vi "Flow.vi"() -> ()   [LabVIEW 2018]
uses:
  <vilib>/Utility/config.llb/Config Data RefNum.ctl
  <vilib>/Utility/sysdir.llb/System Directory Type.ctl
  modules/Serial - XON-XOFF Characters.ctl
  modules/Serial - ASCII Characters.ctl
  modules/Serial - Settings.ctl
  <vilib>/Utility/config.llb/Read Key (String).vi
  <vilib>/Utility/config.llb/Write Key (String).vi
  <vilib>/Utility/config.llb/NI_LVConfig.lvlib
panel:
  out "error out":errorcluster
  out "queue":refnum<queue>
  out "Driver Status":errorcluster
  in  "Marker":string="start_marker"
  out "State":enum16{"Connect", "Acquire", "Standby"}(ring)=enum."Standby"
  in  "S4":dbl[](array[numeric])=[0.0, 0.0, 0.0, 0.0]
  in  "S3":dbl[](array[numeric])=[0.0, 0.0, 0.0, 0.0]
  in  "S2":dbl[](array[numeric])=[0.0, 0.0, 0.0, 0.0]
  in  "S1":dbl[](array[numeric])=[0.0, 0.0, 0.0, 0.0]
  out "System Path":path
  out "dStruct":string[](array[string])
  out "TDMS":refnum<k34>
  in  "?":enum32{"Overview", "Flow vs. Pressure Char"}(tab)
  out "Waveform Chart":dbl(graph)
  out "Flow vs Pressure":cluster{"X":dbl[], "Y":dbl[]}[](graph)
  in  "Enable":bool=TRUE
  in  "Tab Control":enum32{"Connection", "Diagnostic"}(tab)
  in  "add marker":bool
  in  "Record":bool
  in  "New File":bool
  in  "markerString":string
  in  "Folder":path
  in  "File Name":string="database"
  in  "VISA":refnum<visa-resource-name>="COM4"
  in  "EXIT":bool
  in  "Connect":bool
  out "Latency:":dbl
  out "Terminal":string
  in  "Command Terminal":string
  out "Serial Settings:Number of Bytes at Serial Port":u32
  out "Device:":string
  out "Battery Voltage":dbl(slide) scale=3.2..4.2 scale format="%#_2g"
  out "Error Out":errorcluster
  out "Config File":T1
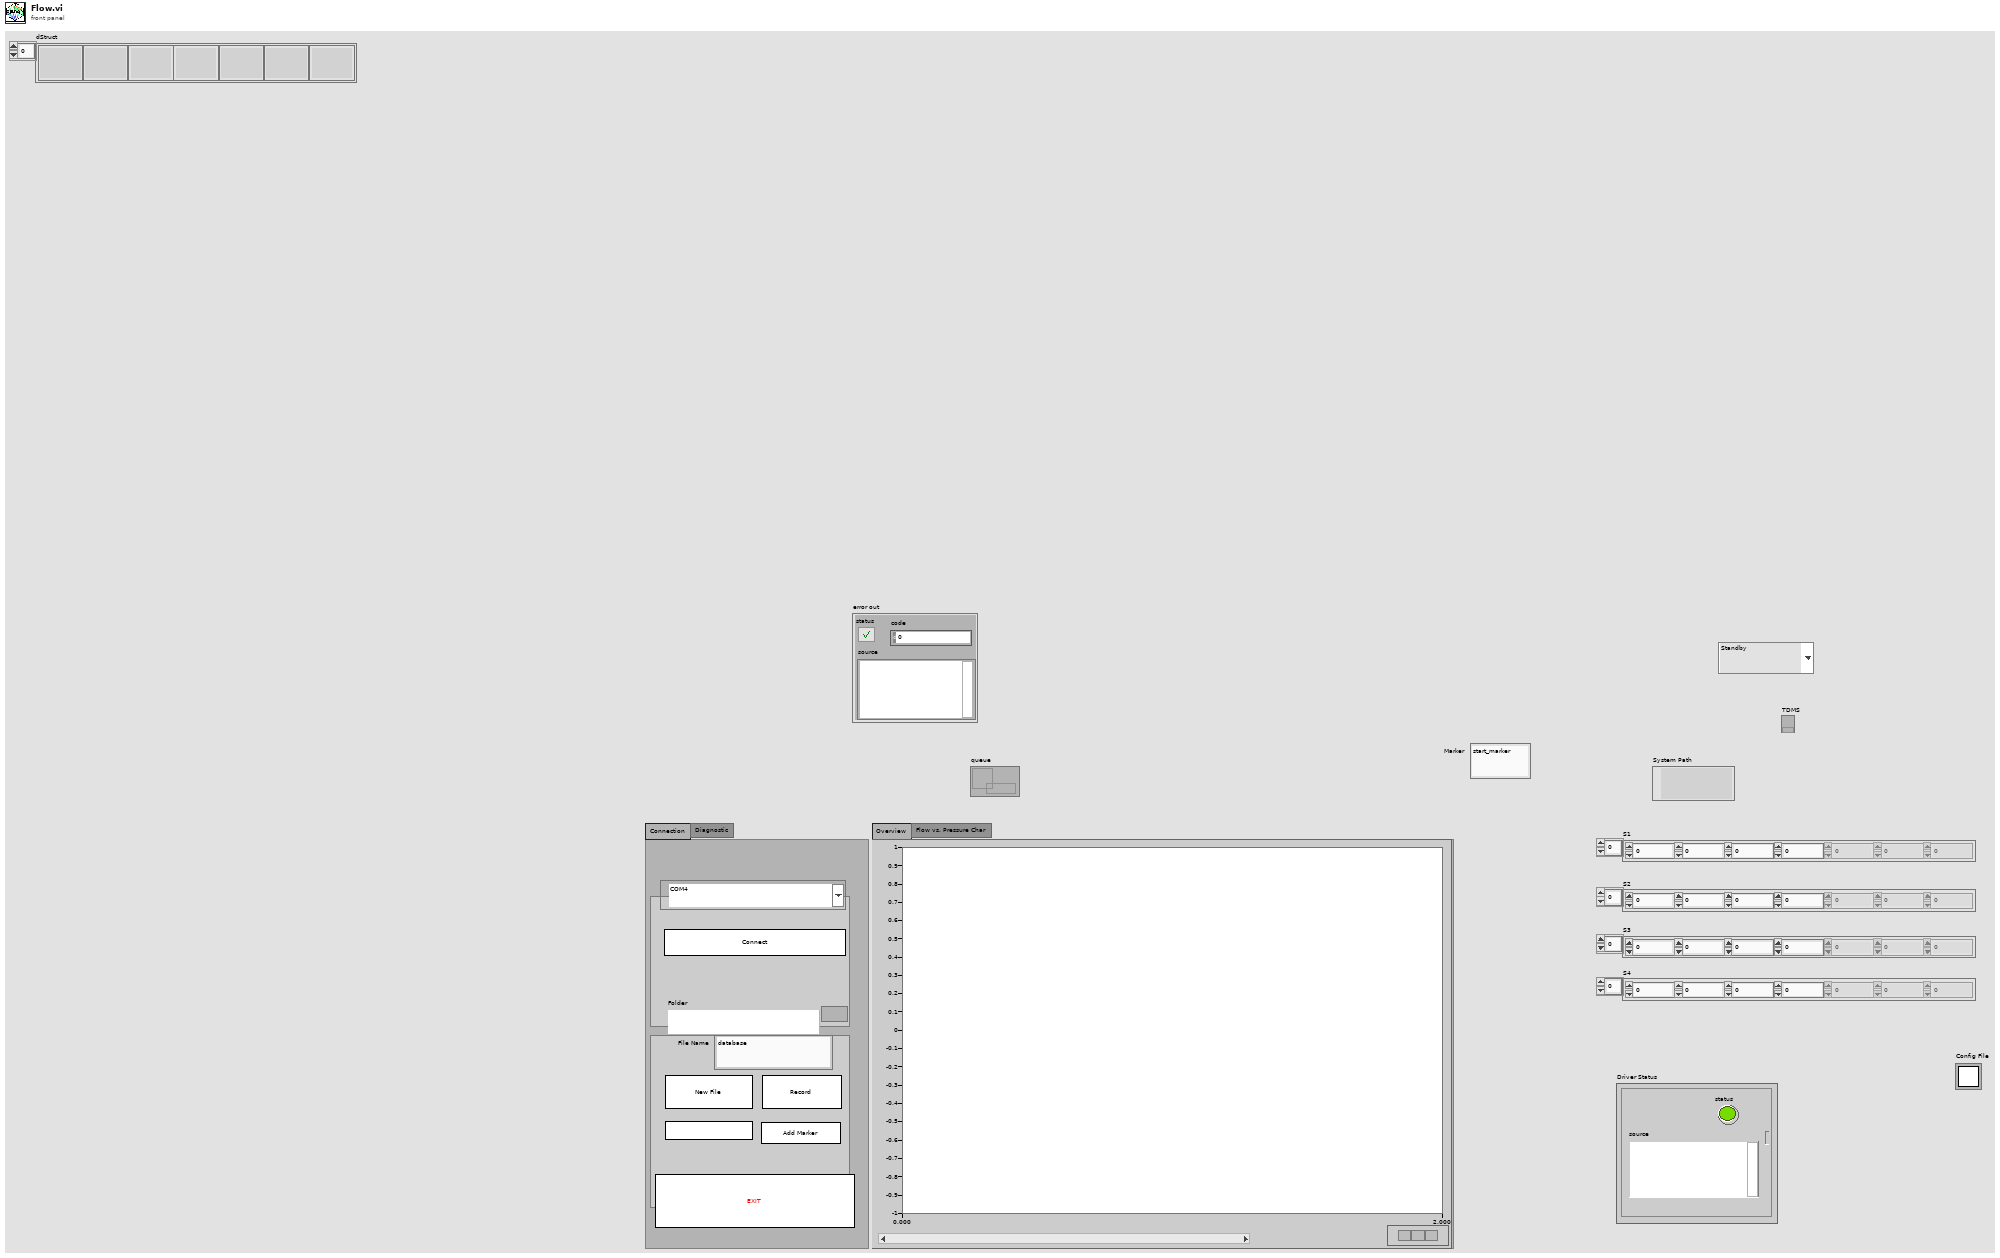
[diagram p1: front panel]
types:
  T1 = typedef "NI_LVConfig.lvlib/Config Data RefNum.ctl" = refnum<k1>
  T2 = cluster{"Dynamic Data Type":dynamicdata, string[]}
  T3 = typedef "System Directory Type.ctl" = i32
  T4 = typedef "Serial - Settings.ctl" = cluster{"baud rate":u32, "data bits":u16, "parity":enum16{"None", "Odd", "Even", "Mark", "Space"}, "stop bits":u16, "flow control":u16}
  T5 = typedef "Serial - XON-XOFF Characters.ctl" = cluster{"XON":T6, "XOFF":T6}
  T6 = typedef "Serial - ASCII Characters.ctl" = enum16{"NUL", "SOH", "STX", "ETX", "EOT", "ENQ", "ACK", "BEL", "BS", "HT", "LF", "VT", "FF", "CR", "SO", "SI", "DLE", "DC1", "DC2", "DC3", "DC4", "NAK", "SYN", "ETB", "CAN", "EM", "SUB", "ESC", "FS", "GS", "RS", "US", "SP", "!", "\"", "#", "$", "%", "&", "'", "(", ")", "*", "+", ",", "- (-)", ".", "/", "0", "1", "2", "3", "4", "5", "6", "7", "8", "9", ":", ";", "<", "=", ">", "?", "@", "A", "B", "C", "D", "E", "F", "G", "H", "I", "J", "K", "L", "M", "N", "O", "P", "Q", "R", "S", "T", "U", "V", "W", "X", "Y", "Z", "[", "\\", "]", "^", "_", "`", "a", "b", "c", "d", "e", "f", "g", "h", "i", "j", "k", "l", "m", "n", "o", "p", "q", "r", "s", "t", "u", "v", "w", "x", "y", "z", "{", "|", "}", "~"}
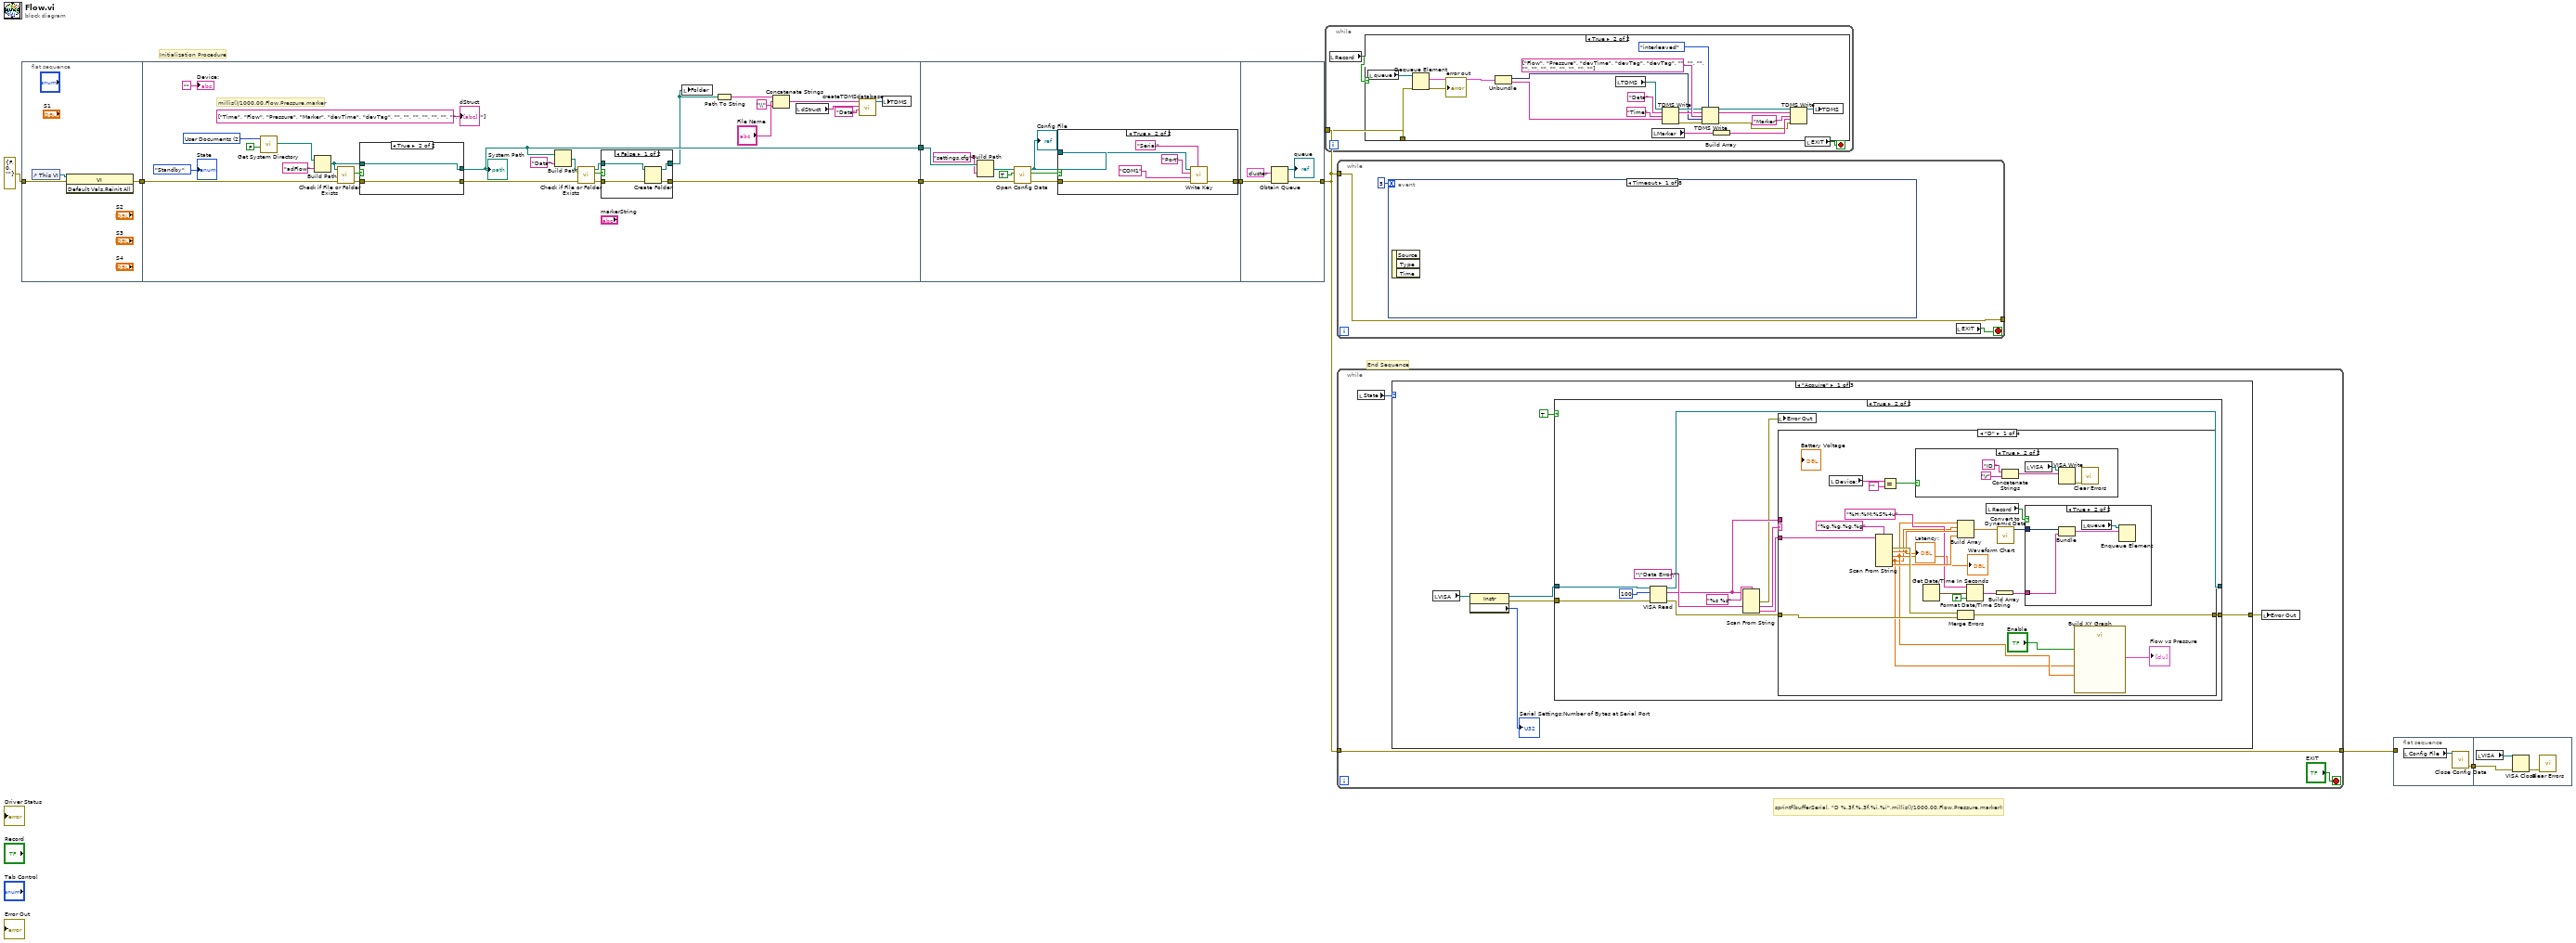
[diagram p0: block diagram]
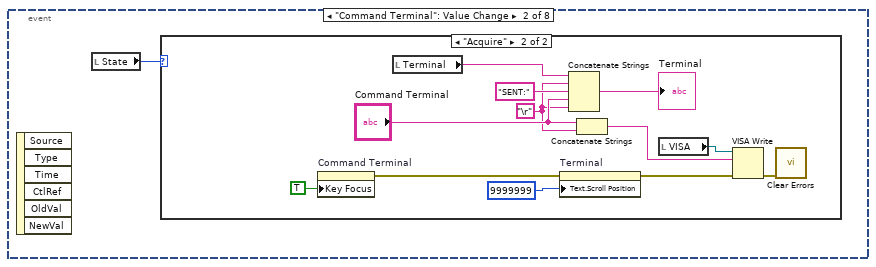
[diagram p3: hidden frame]
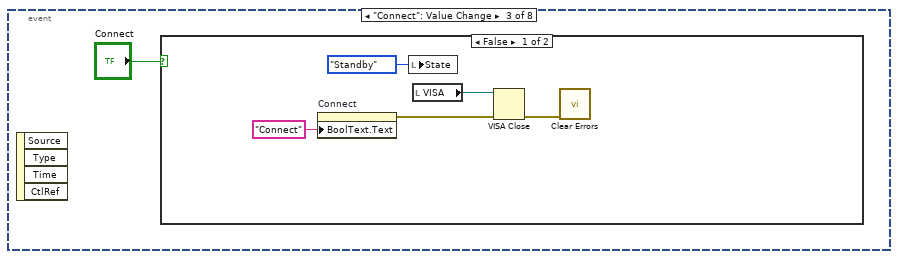
[diagram p5: hidden frame]
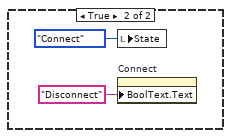
[diagram p6: hidden frame]
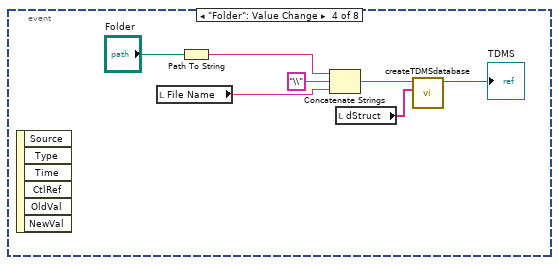
[diagram p7: hidden frame]
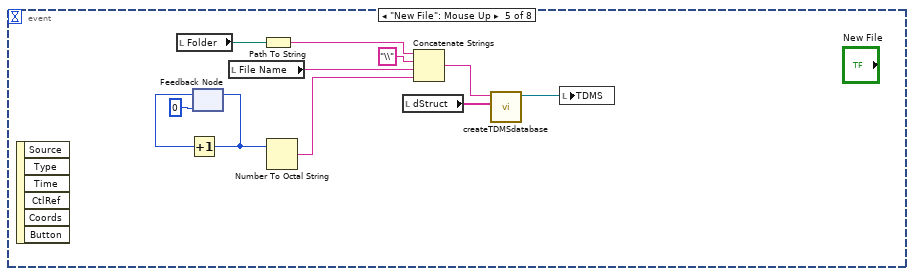
[diagram p8: hidden frame]
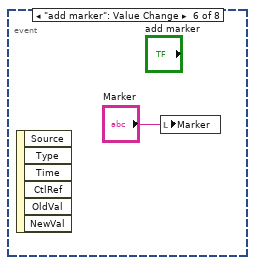
[diagram p9: hidden frame]
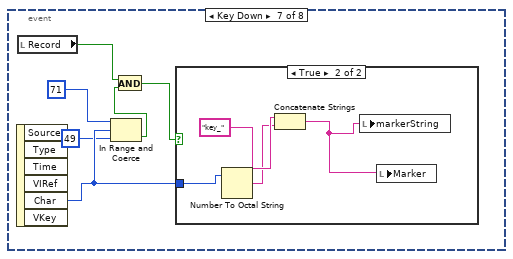
[diagram p10: hidden frame]
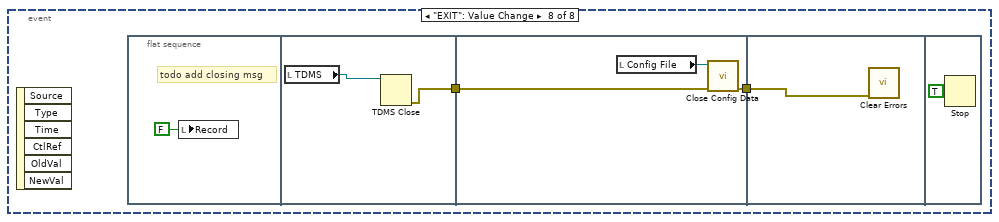
[diagram p12: hidden frame]
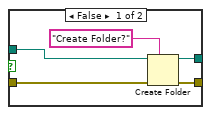
[diagram p14: hidden frame]
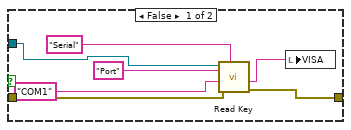
[diagram p15: hidden frame]
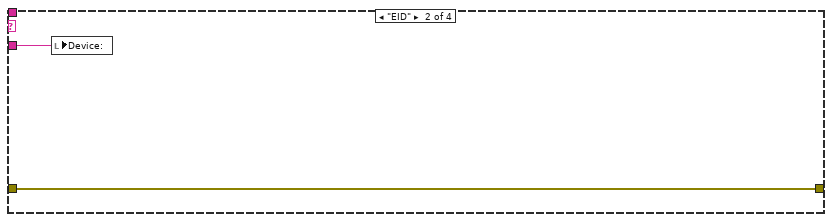
[diagram p19: hidden frame]
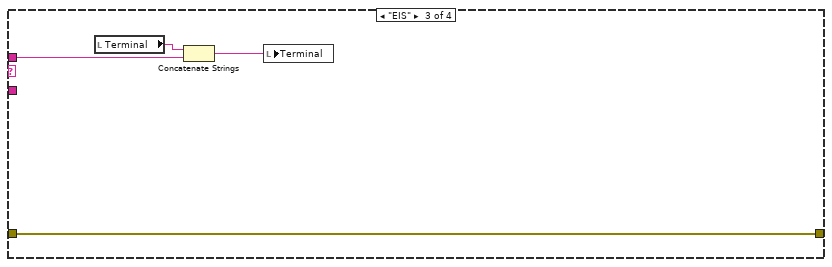
[diagram p20: hidden frame]
diagram:
  # "sprintf(bufferSerial, \"D %.3f,%.3f,%i,%i\",millis()/1000.00,Flow,Pressure,marker);"
  # "End Sequence"
  # "Initialization Procedure"
  n1 = flat-sequence {
    tunnel: errorcluster {"status"=FALSE, "code"=0, "source"=""} ("error in (no error)") -> [w10]
    tunnel: [w9] -> w5
    tunnel: [w28] -> w7
    tunnel: [w25] -> w6
    tunnel: w5 -> [w34]
    tunnel: w7 -> [w58]
    tunnel: w6 -> [w60]
    tunnel: [w52] -> w3
    tunnel: [w75] -> w2
    tunnel: w3 -> [w77]
    frame #0 {
      n2 = control-ref of="This VI"() -> (w11:refnum<vi>)
      n3 = invoke class="VI" method="Default Vals.Reinit All"(reference=w11, error in=w10) -> (error out=w9:errorcluster)  [unwired: 1 in, 2 out]
    }
    frame #1 {
      w37 = T3 2 items=["User Home"=0, "User Desktop"=1, "User Documents"=2, "User Application Data"=3, "User Preferences"=4, "User Temporary"=5, "Public Documents"=6, "Public Application Data"=7, "Public Preferences"=8, "Public Cache"=13, "System Core Libraries"=9, "System Installed Libraries"=10, "Application Files"=11, "Boot Volume Root"=12] ("system directory type")
      # "millis()/1000.00,Flow,Pressure,marker"
      n4 = call <vilib>:"Get System Directory.vi"("create directory if not found? (F)"=FALSE, "system directory type"=w37) -> ("system directory"=w36:path)  [unwired: 9 in]
      n5 = Build Path(base path=w36, name or relative path="adFlow") -> (appended path=w32:path)
      n6 = call <vilib>:"Check if File or Folder Exists.vi"("error in (no error)"=w34, "path"=w32) -> ("error out"=w31:errorcluster, "file or folder exists?"=w33:bool)  [unwired: 7 in, 1 out]
      n7 = case shown="True" w33 {
        tunnel: w32 -> [w49 w51]
        tunnel: w31 -> [w48 w50]
        tunnel: [w46 w51] -> w28
        tunnel: [w45 w50] -> w27
        frame False {
          n8 = Create Folder(prompt (Create Folder)="Create Folder?", path (use dialog)=w49, error in=w48) -> (created path=w46:path, error out=w45:errorcluster)  [unwired: 1 out]
        }
        frame True {
        }
      }
      "System Path" <- w28
      n9 = Build Path(base path=w28, name or relative path="Data") -> (appended path=w29:path)
      n10 = call <vilib>:"Check if File or Folder Exists.vi"("error in (no error)"=w27, "path"=w29) -> ("error out"=w26:errorcluster, "file or folder exists?"=w24:bool, "dup path"=w23:path)  [unwired: 7 in]
      n11 = case shown="False" w24 {
        tunnel: [w41 w44] -> w25
        tunnel: w26 -> [w42 w44]
        tunnel: w23 -> [w40 w43]
        tunnel: [w39 w43] -> w21
        frame False {
          n12 = Create Folder(path (use dialog)=w40, error in=w42) -> (created path=w39:path, error out=w41:errorcluster)  [unwired: 1 in, 1 out]
        }
        frame True {
        }
      }
      n13 = local write "Folder"(w21) -> ()
      n14 = Path To String(path=w21) -> (string=w16:string)
      n15 = Concatenate Strings(w16, "\\" ("string"), "File Name") -> (w20:string)
      n16 = local read "dStruct"() -> (w19:string[])
      n17 = call "createTDMSdatabase.vi"("group name in (Untitled)"="Data", "channel name(s) in (Untitled)"=w19, "String"=w20) -> ("Refnum out"=w22:refnum<k34>)  [unwired: 8 in]
      n18 = local write "TDMS"(w22) -> ()
      "dStruct" <- string[] ["Time", "Flow", "Pressure", "Marker", "devTime", "devTag", "", "", "", "", "", "", "", "", "", ""] ("Channel Names")
      "Device:" <- ""
      "State" <- enum16{"Connect", "Acquire", "Standby"}."Standby" ("State")
    }
    frame #2 {
      n19 = Build Path(base path=w58, name or relative path="settings.cfg") -> (appended path=w56:path)
      n20 = call <vilib>:"Open Config Data.vi"("error in (no error)"=w60, "create file if necessary (T)"=TRUE, "configuration file path"=w56) -> ("error out"=w53:errorcluster, "file created?"=w55:bool, "refnum"=w54:T1)  [unwired: 6 in]
      "Config File" <- w54
      n21 = case shown="True" w55 {
        tunnel: w54 -> [w61 w73]
        tunnel: w53 -> [w63 w72]
        tunnel: [w62 w71] -> w52
        frame False {
          n22 = call-poly <vilib>:"Read Key.vi"("section"="Serial", "error in (no error)"=w63, "default value"="COM1" ("key"), "key"="Port", "refnum"=w61) -> ("error out"=w62:errorcluster, "value"=w67:string)  [unwired: 3 in, 2 out]
          n23 = local write "VISA"(w67) -> ()
        }
        frame True {
          n24 = call-poly <vilib>:"Write Key.vi"("section"="Serial", "error in (no error)"=w72, "value"="COM1" ("key"), "key"="Port", "refnum"=w73) -> ("error out"=w71:errorcluster)  [unwired: 4 in, 2 out]
        }
      }
    }
    frame #3 {
      n25 = Obtain Queue(element data type=T2 {"Dynamic Data Type"=[{"t0"=timestamp(0 s since 1904-01-01), "dt"=1.0, "Y"=[0.0, 0.0, 0.0, 0.0]}, {"t0"=timestamp(3629832558.8844056 s since 1904-01-01), "dt"=1.0, "Y"=[0.0]}, {"t0"=timestamp(3629832558.8844056 s since 1904-01-01), "dt"=1.0, "Y"=[1628.381]}, {"t0"=timestamp(3629832558.8844056 s since 1904-01-01), "dt"=1.0, "Y"=[0.0]}], ["0:00:00.0000"]} ("queue cluster"), error in (no error)=w77) -> (queue out=→"queue":refnum<queue>, error out=w75:errorcluster)  [unwired: 3 in, 1 out]
    }
  }
  n26 = while {
    tunnel: w2 -> [w80]
    stop <- w79 stop-if-true
    n27 = local read "Record"() -> (w78:bool)
    n28 = case shown="True" w78 {
      tunnel: w80 -> [_ w100]
      frame False {
      }
      frame True {
        n29 = local read "queue"() -> (w101:refnum<queue>)
        n30 = Dequeue Element(queue=w101, error in (no error)=w100) -> (element=w99:T2, error out=→"error out":errorcluster)  [unwired: 1 in, 2 out]
        n31 = Unbundle(w99) -> ("Dynamic Data Type"=w83:dynamicdata, w84:string[])
        n32 = local read "TDMS"() -> (w92:refnum<k34>)
        n33 = local read "Marker"() -> (w93:string)
        n34 = TDMS Write(0:w92, 5:"Data" ("group name in (Untitled)"), 7:"Time" ("group name in (Untitled)"), 9:w84) -> (4:w88:refnum<k34>, 6:w89:string, 15:w90:errorcluster)  [unwired: 2 in, 1 out]
        n35 = TDMS Write(0:w88, 1:enum16{"decimated", "interleaved"}."interleaved" ("data layout (0:decimated)"), 5:w89, 7:string[] ["Flow", "Pressure", "devTime", "devTag", "devTag", "", "", "", "", "", "", "", "", "", "", ""] ("Channel Names"), 9:w83, 11:w90) -> (4:w86:refnum<k34>, 6:w85:string, 15:w81:errorcluster)  [unwired: 1 out]
        n36 = Build Array(w93) -> (w94:string[])
        n37 = TDMS Write(0:w86, 5:w85, 7:"Marker" ("channel name(s) in (Untitled)"), 9:w94, 11:w81) -> (4:w97:refnum<k34>)  [unwired: 1 in, 3 out]
        n38 = local write "TDMS"(w97) -> ()
      }
    }
    n39 = local read "EXIT"() -> (w79:bool)
  }
  n40 = while {
    tunnel: w2 -> [w103]
    tunnel: [w103] -> _
    stop <- w104 stop-if-true
    n41 = event shown="[0] Timeout" {
      selector: _ -> [_ _ _ _ _ _ _ _]
      dyn-events: _ -> [_ _ _ _ _ _ _ _]
      timeout: 5 -> [_ _ _ _ _ _ _ _]
      event Timeout {
        n42 = event-data() -> ()  [unwired: 1 in, 3 out]
      }
      event "Command Terminal": Value Change {
        n43 = event-data() -> ()  [unwired: 1 in, 6 out]
        n44 = local read "State"() -> (w105:enum16{"Connect", "Acquire", "Standby"})
        n45 = case shown="\"Acquire\"" w105 {
          frame "Connect", Default {
          }
          frame "Acquire" {
            w108 = "\r"
            n46 = property on="Command Terminal" class="Str"("Key Focus"=TRUE) -> (error out=w113:errorcluster)  [unwired: 2 in, 1 out]
            n47 = local read "Terminal"() -> (w117:string)
            n48 = property on="Terminal" class="Str"(error in=w113, "Text.Scroll Position"=u32 9999999) -> (error out=w109:errorcluster)  [unwired: 1 in, 1 out]
            n49 = Concatenate Strings(w117, w108, "SENT:" ("string"), "Command Terminal", w108) -> (→"Terminal":string)
            n50 = Concatenate Strings("Command Terminal", w108) -> (w110:string)
            n51 = local read "VISA"() -> (w107:refnum<visa-resource-name>)
            n52 = VISA Write(VISA resource name=w107, write buffer=w110, error in (no error)=w109) -> (error out=w106:errorcluster)  [unwired: 2 out]
            n53 = call <vilib>:"Clear Errors.vi"("error in (no error)"=w106) -> ()  [unwired: 5 in, 2 out]
          }
        }
      }
      event "Connect": Value Change {
        n54 = event-data() -> ()  [unwired: 1 in, 4 out]
        n55 = case shown="False" "Connect" {
          frame False {
            n56 = property on="Connect" class="Bool (strict)"("BoolText.Text"="Connect" ("Boolean Text.Text")) -> (error out=w121:errorcluster)  [unwired: 2 in, 1 out]
            n57 = local write "State"(enum16{"Connect", "Acquire", "Standby"}."Standby" ("Enum")) -> ()
            n58 = local read "VISA"() -> (w120:refnum<visa-resource-name>)
            n59 = VISA Close(VISA resource name=w120, error in (no error)=w121) -> (error out=w119:errorcluster)
            n60 = call <vilib>:"Clear Errors.vi"("error in (no error)"=w119) -> ()  [unwired: 5 in, 2 out]
          }
          frame True {
            n61 = local write "State"(enum16{"Connect", "Acquire", "Standby"}."Connect" ("Enum")) -> ()
            n62 = property on="Connect" class="Bool (strict)"("BoolText.Text"="Disconnect" ("Boolean Text.Text")) -> ()  [unwired: 2 in, 2 out]
          }
        }
      }
      event "Folder": Value Change {
        n63 = event-data() -> ()  [unwired: 1 in, 6 out]
        n64 = local read "File Name"() -> (w127:string)
        n65 = Path To String(path="Folder") -> (string=w129:string)
        n66 = Concatenate Strings(w129, "\\" ("string"), w127) -> (w126:string)
        n67 = local read "dStruct"() -> (w130:string[])
        n68 = call "createTDMSdatabase.vi"("channel name(s) in (Untitled)"=w130, "String"=w126) -> ("Refnum out"=→"TDMS":refnum<k34>)  [unwired: 9 in]
      }
      event "New File": Mouse Up {
        n69 = event-data() -> ()  [unwired: 1 in, 6 out]
        n70 = local read "Folder"() -> (w140:path)
        n71 = feedback #1(0) -> (w141:i32)
        n72 = Increment(x=w141) -> (x+1=w143:i32)
        n73 = feedback-in #1(w143) -> ()
        n74 = local read "File Name"() -> (w134:string)
        n75 = Path To String(path=w140) -> (string=w136:string)
        n76 = Number To Octal String(2:w143) -> (0:w133:string)  [unwired: 1 in]
        n77 = local read "dStruct"() -> (w137:string[])
        n78 = Concatenate Strings(w136, "\\" ("string"), w134, w133) -> (w139:string)
        n79 = call "createTDMSdatabase.vi"("channel name(s) in (Untitled)"=w137, "String"=w139) -> ("Refnum out"=w138:refnum<k34>)  [unwired: 9 in]
        n80 = local write "TDMS"(w138) -> ()
      }
      event "add marker": Value Change {
        n81 = event-data() -> ()  [unwired: 1 in, 6 out]
        n82 = local write "Marker"("Marker") -> ()
      }
      event Key Down {
        n83 = event-data() -> ("Char"=w150:i16)  [unwired: 1 in, 5 out]
        n84 = local read "Record"() -> (w148:bool)
        n85 = In Range and Coerce(upper limit=i16 71, x=w150, lower limit=i16 49) -> (In Range?=w146:bool)  [unwired: 1 out]
        n86 = And(x=w148, y=w146) -> (x .and. y?=w145:bool)
        n87 = case shown="True" w145 {
          tunnel: w150 -> [_ w151]
          frame False {
          }
          frame True {
            n88 = Number To Octal String(2:w151) -> (0:w153:string)  [unwired: 1 in]
            n89 = Concatenate Strings("key_" ("element"), w153) -> (w152:string)
            n90 = local write "markerString"(w152) -> ()
            n91 = local write "Marker"(w152) -> ()
          }
        }
      }
      event "EXIT": Value Change {
        n92 = event-data() -> ()  [unwired: 1 in, 6 out]
        n93 = flat-sequence {
          tunnel: [w158] -> w155
          tunnel: [w161] -> w156
          tunnel: w155 -> [w160]
          tunnel: w156 -> [w163]
          frame #0 {
            # "todo add closing msg"
            n94 = local write "Record"(FALSE ("Record")) -> ()
          }
          frame #1 {
            n95 = local read "TDMS"() -> (w159:refnum<k34>)
            n96 = TDMS Close(11:w159) -> (0:w158:errorcluster)  [unwired: 1 in, 1 out]
          }
          frame #2 {
            n97 = local read "Config File"() -> (w162:T1)
            n98 = call <vilib>:"Close Config Data.vi"("error in (no error)"=w160, "refnum"=w162) -> ("error out"=w161:errorcluster)  [unwired: 8 in, 1 out]
          }
          frame #3 {
            n99 = call <vilib>:"Clear Errors.vi"("error in (no error)"=w163) -> ()  [unwired: 5 in, 2 out]
          }
          frame #4 {
            n100 = Stop(stop? (T)=TRUE) -> ()
          }
        }
      }
    }
    n101 = local read "EXIT"() -> (w104:bool)
  }
  n102 = while {
    tunnel: w2 -> [w167]
    tunnel: [w167] -> w4
    stop <- "EXIT" stop-if-true
    n103 = local read "State"() -> (w166:enum16{"Connect", "Acquire", "Standby"})
    n104 = case shown="\"Acquire\"" w166 {
      tunnel: [w174 errorcluster {"status"=FALSE, "code"=0, "source"=""} ("error out") w229] -> w165
      frame "Acquire" {
        n105 = local read "VISA"() -> (w170:refnum<visa-resource-name>)
        n106 = property class="Instr"(reference=w170) -> (reference out=w172:refnum<visa-resource-name>, error out=w173:errorcluster, "Serial Settings:Number of Bytes at Serial Port"=→"Serial Settings:Number of Bytes at Serial Port":u32)  [unwired: 1 in]
        n107 = case shown="True" TRUE {
          tunnel: [w176 w183] -> w174
          tunnel: w173 -> [w176 w188]
          tunnel: w172 -> [w175 w187]
          tunnel: [w175 w186] -> _
          frame False {
          }
          frame True {
            n108 = VISA Read(VISA resource name=w187, byte count=u32 100, error in (no error)=w188) -> (VISA resource name out=w186:refnum<visa-resource-name>, read buffer=w179:string, error out=w184:errorcluster)  [unwired: 1 out]
            n109 = Scan From String(format string="%s %s", input string=w179, default 1="\"Data Error\"" ("default value 1")) -> (error out=w178:errorcluster, output 1=w180:string, output 2=w177:string)  [unwired: 3 in, 2 out]
            n110 = local write "Error Out"(w178) -> ()
            n111 = case shown="\"D\"" w180 {
              tunnel: w184 -> [w209 w221 w223 w226]
              tunnel: [w207 w221 w223 w226] -> w183
              tunnel: w179 -> [_ _ w222 _]
              tunnel: w177 -> [w199 w220 _ _]
              frame "D" {
                n112 = local read "Device:"() -> (w204:string)
                n113 = Scan From String(format string="%g,%g,%g,%g", input string=w199) -> (error out=w208:errorcluster, output 1=w198:dbl, output 2=w191:dbl, output 3=w190:dbl, output 4=w201:dbl)  [unwired: 6 in, 2 out]
                "Waveform Chart" <- w191
                "Latency:" <- w198
                n114 = Equal?(x=w204, y="") -> (x = y?=w203:bool)
                n115 = case shown="True" w203 {
                  frame False {
                  }
                  frame True {
                    n116 = Concatenate Strings("ID " ("string"), "\r") -> (w215:string)
                    n117 = local read "VISA"() -> (w212:refnum<visa-resource-name>)
                    n118 = VISA Write(VISA resource name=w212, write buffer=w215) -> (error out=w211:errorcluster)  [unwired: 1 in, 2 out]
                    n119 = call <vilib>:"Clear Errors.vi"("error in (no error)"=w211) -> ()  [unwired: 5 in, 2 out]
                  }
                }
                n120 = Get Date/Time In Seconds() -> (seconds since 1Jan1904=w196:timestamp)
                n121 = Build Array(w191, w190, w198, w201) -> (w205:dbl[])
                n122 = Merge Errors(w208, w209) -> (w207:errorcluster)
                n123 = Format Date/Time String(time format string (%c)="%H:%M:%S%4u", seconds (now)=w196, UTC format=FALSE) -> (date/time string=w195:string)
                n124 = local read "Record"() -> (w206:bool)
                n125 = Build Array(w195) -> (w193:string[])
                n126 = call "Convert to Dynamic Data"("Array"=w205) -> ("Dynamic Data Type"=w200:dynamicdata)  [unwired: 3 in]
                n127 = case shown="True" w206 {
                  tunnel: w200 -> [_ w219]
                  tunnel: w193 -> [_ w218]
                  frame False {
                  }
                  frame True {
                    n128 = Bundle("Dynamic Data Type"=w219, w218) -> (w217:T2)  [unwired: 1 in]
                    n129 = local read "queue"() -> (w216:refnum<queue>)
                    n130 = Enqueue Element(queue=w216, element=w217) -> ()  [unwired: 2 in, 3 out]
                  }
                }
                n131 = call "Build XY Graph"("Enable"="Enable", "Y Input"=w191, "X Input"=w190) -> ("XY Graph"=→"Flow vs Pressure":cluster{"X":dbl[], "Y":dbl[]}[])  [unwired: 7 in, 1 out]
              }
              frame "EID" {
                n132 = local write "Device:"(w220) -> ()
              }
              frame "EIS" {
                n133 = local read "Terminal"() -> (w224:string)
                n134 = Concatenate Strings(w224, w222) -> (w225:string)
                n135 = local write "Terminal"(w225) -> ()
              }
              frame "Data Error", Default {
              }
            }
          }
        }
      }
      frame "Standby", Default {
      }
      frame "Connect" {
        n136 = call "open_serial.vi"("End Write on Termination Character?"=TRUE, "XON/XOFF Characters"=T5 {"XON"=enum."DC1", "XOFF"=enum."DC3"}, "Termination Character"=u8 10, "Serial Settings"=T4 {"baud rate"=9600, "data bits"=8, "parity"=enum."None", "stop bits"=10, "flow control"=0}, "End Read on Termination Character?"=TRUE, "VISA Refnum in"="VISA") -> ("error out"=w231:errorcluster)  [unwired: 4 in, 1 out]
        n137 = call <vilib>:"Clear Errors.vi"("error in (no error)"=w231) -> ("error out"=w228:errorcluster)  [unwired: 5 in, 1 out]
        n138 = case shown="No Error" w228 {
          selector: w228 -> [w240 w244]
          tunnel: [w239 w244] -> w229
          frame No Error {
            n139 = local read "Config File"() -> (w237:T1)
            n140 = local read "VISA"() -> (w238:refnum<visa-resource-name>)
            n141 = call-poly <vilib>:"Write Key.vi"("section"="Serial", "error in (no error)"=w240, "value"=w238, "key"="Port", "refnum"=w237) -> ("error out"=w239:errorcluster)  [unwired: 4 in, 2 out]
            n142 = local write "State"(enum16{"Connect", "Acquire", "Standby"}."Acquire" ("Enum")) -> ()
          }
          frame Error {
            n143 = local read "VISA"() -> (w246:refnum<visa-resource-name>)
            n144 = property on="Connect" class="Bool (strict)"("Value"=FALSE ("Connect")) -> ()  [unwired: 2 in, 2 out]
            n145 = VISA Close(VISA resource name=w246) -> (error out=w245:errorcluster)  [unwired: 1 in]
            n146 = call <vilib>:"Clear Errors.vi"("error in (no error)"=w245) -> ()  [unwired: 5 in, 2 out]
            n147 = local write "State"(enum16{"Connect", "Acquire", "Standby"}."Standby" ("Enum")) -> ()
          }
        }
      }
    }
    n148 = local write "Error Out"(w165) -> ()
  }
  n149 = flat-sequence {
    tunnel: w4 -> [_]
    tunnel: [w249] -> w1
    tunnel: w1 -> [w251]
    frame #0 {
      n150 = local read "Config File"() -> (w250:T1)
      n151 = call <vilib>:"Close Config Data.vi"("refnum"=w250) -> ("error out"=w249:errorcluster)  [unwired: 9 in, 1 out]
    }
    frame #1 {
      n152 = local read "VISA"() -> (w252:refnum<visa-resource-name>)
      n153 = VISA Close(VISA resource name=w252, error in (no error)=w251) -> (error out=w253:errorcluster)
      n154 = call <vilib>:"Clear Errors.vi"("error in (no error)"=w253) -> ()  [unwired: 5 in, 2 out]
    }
  }
